vi "Panel Resend Start.vi"(0 "Enable":bool=TRUE, 5 "error in (no error)":errorcluster, 6 "All Confgured Com Array":u8[](array[numeric])=[100, 2, 3, 4, 5, 6, 7, 8, 9, 10, 11, 12, 13, 14, 15, 16, 17, 18, 19, 20, 21, 22, 23, 24, 25, 26, 27, 28, 29, 30, 31, 32, 33, 34, 35, 36, 37, 38, 39, 40, 41, 42, 43, 44, 45, 46, 47, 48, 49, 50, 51, 52, 53, 54, 55, 56], 8 "Station Labels":string[](array[string])) -> (17 "Com Port":dbl, 18 "Resend":bool, 19 "error out":errorcluster)   [LabVIEW 2012]
doc: "Displays a standard dialog box that prompts users to enter information, such as a user name and password.\n--------------------\n\nThis Express VI is configured as follows:\n\nMessage to Display to the User:\nThe inputs are: \nNumber: Com Port"
panel:
  in  "Station Label":dbl(ring) items=["A"=100.0, "b"=2.0, "c"=3.0, "d"=4.0]
  out "String":string
  in  "Cancel":bool
  in  "OK2":bool
  in  "OK1":bool
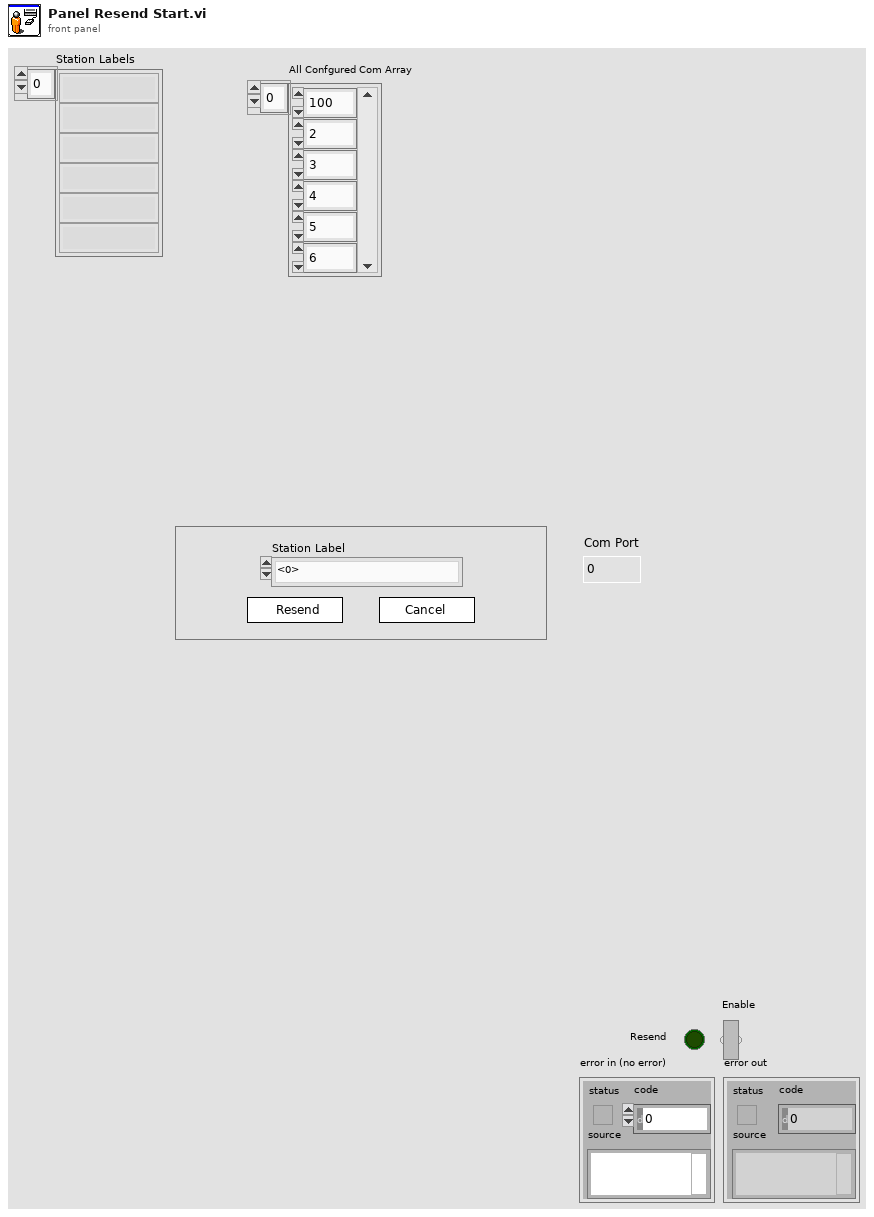
[diagram p1: front panel]
types:
  T1 = cluster{"Input Name":string, "Input Data Type":i32}[]
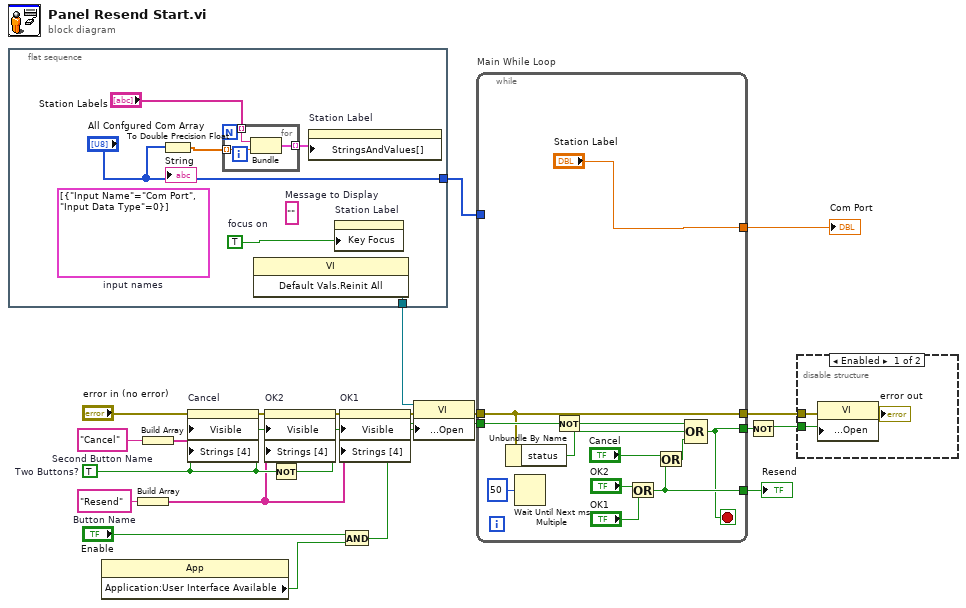
[diagram p0: block diagram]
diagram:
  w13 = "Cancel"  # Second Button Name
  w11 = "Resend"  # Button Name
  w21 = TRUE  # Two Buttons?
  n1 = flat-sequence {
    tunnel: [w27] -> w3
    tunnel: ["All Confgured Com Array"] -> w1
    frame #0 {
      (unwired) T1 [{"Input Name"="Com Port", "Input Data Type"=0}]  # input names
      w22 = TRUE  # focus on
      (unwired) ""  # Message to Display
      n2 = To Double Precision Float(number="All Confgured Com Array") -> (double precision float=w24:dbl[])
      n3 = for {
        tunnel: "Station Labels" -> [w30] mode=indexing
        tunnel: w24 -> [w29] mode=indexing
        tunnel: [w28] -> w23 mode=indexing
        n4 = Bundle(w30, "Start Com Chan"=w29) -> (w28:cluster{string, "Start Com Chan":dbl})  [unwired: 1 in]
      }
      n5 = invoke class="VI" method="Default Vals.Reinit All"() -> (reference out=w27:refnum<vi>)  [unwired: 3 in, 2 out]
      n6 = property on="Station Label" class="Ring (strict)"("StringsAndValues[]"=w23) -> ()  [unwired: 2 in, 2 out]
      n7 = property on="Station Label" class="Ring (strict)"("Key Focus"=w22) -> ()  [unwired: 2 in, 2 out]
    }
  }
  n8 = property class="App"() -> ("Application:User Interface Available"=w4:bool)  [unwired: 2 in, 2 out]
  n9 = Build Array(w11) -> (w12:string[])
  n10 = Build Array(w13) -> (w14:string[])
  n11 = property on="Cancel" class="Bool"(error in="error in (no error)", "Visible"=w21, "Strings [4]"=w14) -> (error out=w18:errorcluster)  [unwired: 1 in, 1 out]
  n12 = property on="OK2" class="Bool"(error in=w18, "Visible"=w21, "Strings [4]"=w12) -> (error out=w17:errorcluster)  [unwired: 1 in, 1 out]
  n13 = Not(x=w21) -> (.not. x?=w19:bool)
  n14 = property on="OK1" class="Bool"(error in=w17, "Visible"=w19, "Strings [4]"=w12) -> (error out=w10:errorcluster)  [unwired: 1 in, 1 out]
  n15 = And(x="Enable", y=w4) -> (x .and. y?=w5:bool)
  n16 = property class="VI"(reference=w3, error in=w10, "Front Panel Window:Open"=w5) -> (error out=w9:errorcluster)  [unwired: 1 out]
  n17 = while "Main While Loop" {
    tunnel: [w39] -> w20
    tunnel: w5 -> [w37]
    tunnel: [w35] -> w15
    tunnel: w9 -> [w34]
    tunnel: [w34] -> w7
    tunnel: ["Station Label"] -> w2
    tunnel: w1 -> [_]
    stop <- w35 stop-if-true
    n18 = Unbundle By Name(w34) -> ("status"=w32:bool)
    n19 = Wait Until Next ms Multiple(millisecond multiple=u32 50) -> ()  [unwired: 1 out]
    n20 = Not(x=w37) -> (.not. x?=w36:bool)
    n21 = Or(x="OK2", y="OK1") -> (x .or. y?=w39:bool)
    n22 = Or(x="Cancel", y=w39) -> (x .or. y?=w33:bool)
    n23 = Compound Arithmetic op=OR(w36, w32, w33) -> (w35:bool)
  }
  "Resend" <- w20
  "Com Port" <- w2
  n24 = Not(x=w15) -> (.not. x?=w16:bool)
  n25 = disable-structure shown="Enabled" {
    disable-tunnel: w16 -> [w45 _]
    disable-tunnel: w7 -> [w44 _]
    frame Enabled {
      n26 = property class="VI"(error in=w44, "Front Panel Window:Open"=w45) -> (error out=→"error out":errorcluster)  [unwired: 1 in, 1 out]
    }
    frame Disabled {
    }
  }
